vi "HomeStageDll.vi"(8 "error in":errorcluster, 9 "Stage":T1, 11 "DevRefIn":u32) -> (0 "error out":errorcluster, 2 "result string":string, 3 "DevRefOut":u32)   [LabVIEW 2020]
uses:
  StageSelector--Enum.ctl
  gclib32.lvlib
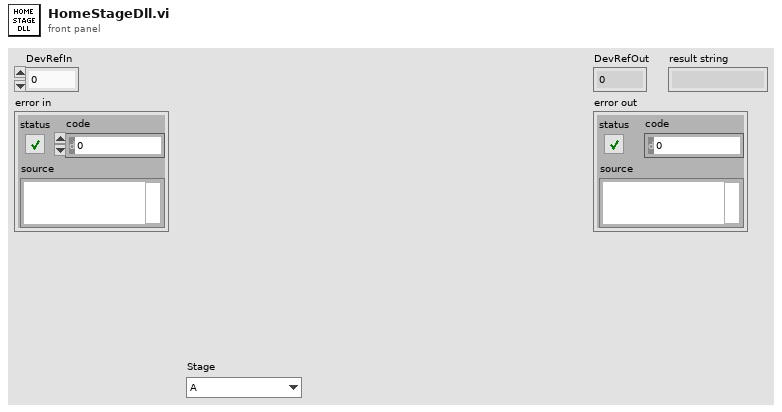
[diagram p1: front panel]
types:
  T1 = typedef "StageSelector--Enum.ctl" = enum16{"A", "B", "C", "D"}
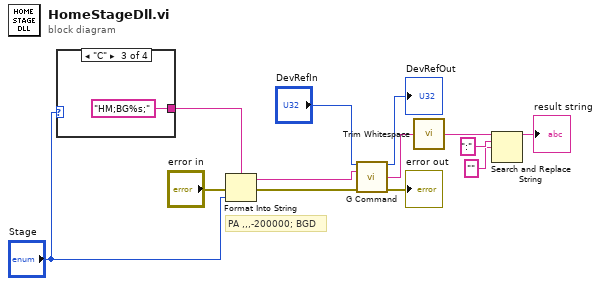
[diagram p0: block diagram]
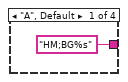
[diagram p2: hidden frame]
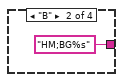
[diagram p3: hidden frame]
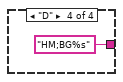
[diagram p4: hidden frame]
diagram:
  # "PA ,,,-200000; BGD"
  n1 = case shown="\"C\"" "Stage" {
    tunnel: ["HM;BG%s" ("format string") "HM;BG%s" ("format string") "HM;BG%s;" ("format string") "HM;BG%s" ("format string")] -> w13
    frame "A", Default {
    }
    frame "B" {
    }
    frame "C" {
    }
    frame "D" {
    }
  }
  n2 = Format Into String(format string=w13, error in="error in", "Stage") -> (resulting string=w3:string, error out=w6:errorcluster)  [unwired: 1 in]
  n3 = call "G Command.vi"("g"="DevRefIn", "command"=w3, "error in (no error)"=w6) -> ("g out"=→"DevRefOut":u32, "buffer out"=w4:string, "error out"=→"error out":errorcluster)  [unwired: 10 in]
  n4 = call "Trim Whitespace.vi"("string"=w4) -> ("trimmed string"=w11:string)  [unwired: 1 in]
  n5 = Search and Replace String(input string=w11, search string=":", replace string="" ("replace string (\"\")")) -> (result string=→"result string":string)  [unwired: 5 in, 3 out]
